vi "Get Connection Status.vi"(8 "error in (no error)":errorcluster, 11 "IP Connection in":refnum<class "IP Connection.lvclass">) -> (0 "error out":errorcluster, 1 "connected?":bool, 2 "Connection Status":T1, 3 "IP Connection out":refnum<class "IP Connection.lvclass">)   [LabVIEW 2011, in "Tinkerforge.lvlib" / "IP Connection.lvclass"]
doc: "This VI returns the connection status of the IP Connection."
uses:
  IP Connection.lvclass
  Type Definitions/Connection Status.ctl
  IP Connection.lvclass/IP Connection.ctl
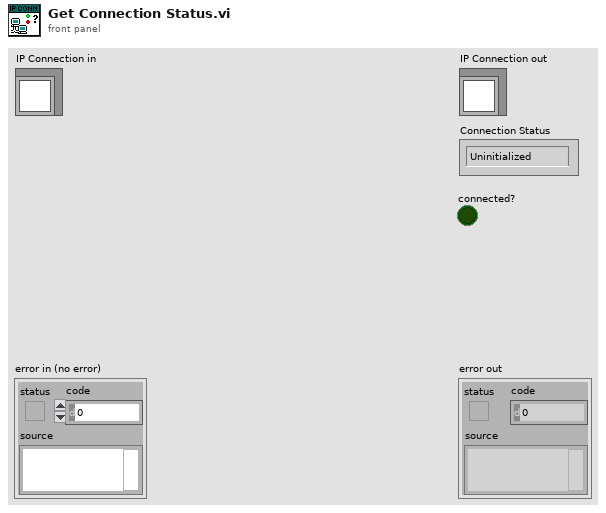
[diagram p1: front panel]
types:
  T1 = typedef "Tinkerforge.lvlib/IP Connection.lvclass/Connection Status.ctl" = enum16{"Uninitialized", "Connected", "Reconnecting", "Disconnected"}
  T2 = typedef "Tinkerforge.lvlib/IP Connection.lvclass/Connection.ctl" = cluster{"TCP Network Connection":refnum<k5>, "is connected":bool, "Connection Status":T1}
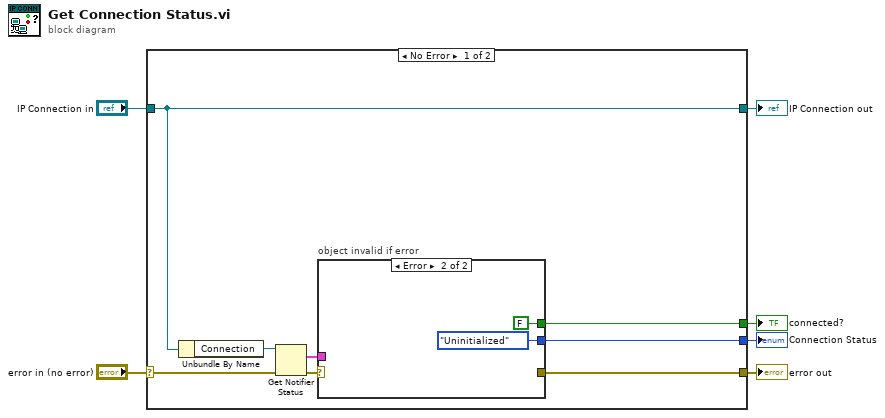
[diagram p0: block diagram]
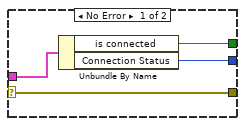
[diagram p2: hidden frame]
diagram:
  n1 = case shown="No Error" "error in (no error)" {
    selector: "error in (no error)" -> [w14 w22]
    tunnel: [w7 w22] -> w5
    tunnel: [w13 w21] -> w3
    tunnel: "IP Connection in" -> [w13 w21]
    tunnel: [w10 _] -> w2
    tunnel: [w9 _] -> w1
    frame No Error {
      n2 = Unbundle By Name(w13) -> ("Connection"=w12:refnum<notifier>)
      n3 = Get Notifier Status(notifier=w12, error in (no error)=w14) -> (current notification=w11:T2, error out=w8:errorcluster)  [unwired: 3 out]
      n4 = case "object invalid if error" shown="Error" w8 {
        selector: w8 -> [w15 _]
        tunnel: w11 -> [w18 _]
        tunnel: [w17 FALSE ("is connected")] -> w10
        tunnel: [w16 Connection_Status."Uninitialized" ("Connection Status")] -> w9
        tunnel: [w15 _] -> w7
        frame No Error {
          n5 = Unbundle By Name(w18) -> ("is connected"=w17:bool, "Connection Status"=w16:T1)
        }
        frame Error {
        }
      }
    }
    frame Error {
    }
  }
  "error out" <- w5
  "IP Connection out" <- w3
  "connected?" <- w2
  "Connection Status" <- w1
